vi "DSF.Engine.Memory.Cache.Transfer.Get Configuration.vi"(11 "Transfer Cache in":refnum<class "DSF.Engine.Memory.Cache.Transfer.lvclass">) -> (2 "Transfer Configuration":refnum<class "DSF.Shared.Configuration.Transfer.lvclass">, 3 "Transfer Cache out":refnum<class "DSF.Engine.Memory.Cache.Transfer.lvclass">)   [LabVIEW 2017, in "DSF.Engine.lvlib" / "DSF.Engine.Memory.Cache.Transfer.lvclass"]
uses:
  DSF.Engine.Memory.Cache.Transfer.lvclass
  Shared/Classes/Transfer/DSF.Shared.Configuration.Transfer.lvclass
  DSF.Engine.Memory.Cache.Transfer.lvclass/DSF.Engine.Memory.Cache.Transfer.ctl
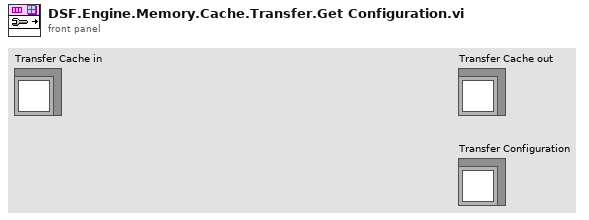
[diagram p1: front panel]
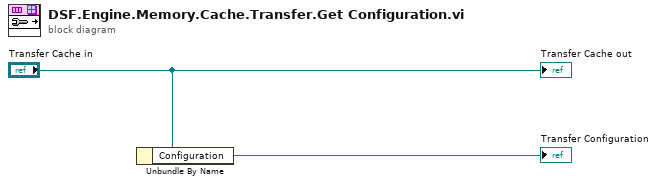
[diagram p0: block diagram]
diagram:
  n1 = Unbundle By Name("Transfer Cache in") -> ("Configuration"=→"Transfer Configuration":refnum<class "DSF.Shared.Configuration.Transfer.lvclass">)
  "Transfer Cache out" <- "Transfer Cache in"
